vi "IMP Panel.vi"(7 "IMP Command":T1, 8 "error in (no error)":errorcluster, 11 "Variant Input":variant) -> (0 "error out":errorcluster, 3 "Variant Output":variant)   [LabVIEW 2011]
uses:
  IMP Command.ctl
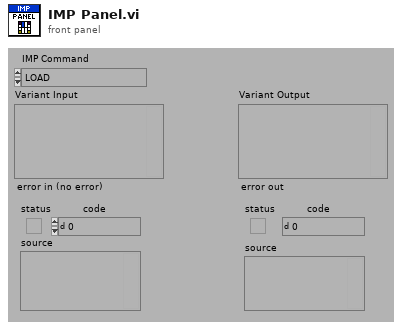
[diagram p1: front panel]
types:
  T1 = typedef "IMP Command.ctl" = enum16{"LOAD", "INITIALIZE", "IMPORT", "UNLOAD"}
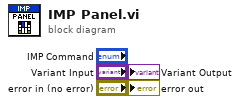
[diagram p0: block diagram]
diagram:
